vi "Log Result.vi"(8 "error in (no error)":errorcluster, 10 "Result":refnum<class "Acquired Result.lvclass">, 11 "Process Controller in":refnum<class "Process Controller.lvclass">) -> (0 "error out":errorcluster, 2 "Result out":refnum<class "Acquired Result.lvclass">, 3 "Process Controller out":refnum<class "Process Controller.lvclass">)   [LabVIEW 2016, in "Process Controller.lvclass"]
uses:
  Process Controller.lvclass
  C:/github/LabActor/Template Module/Template Module.lvclass
  C:/github/LabActor/Worker/Worker.lvclass
  NHMFL_Core/Libraries/Instruments/Results/Acquired Result/Acquired Result.lvclass
  Template Module/Template Module.lvclass/Template Module.ctl
  Process Controller.lvclass/Process Controller.ctl
  Worker/Worker.lvclass/Worker.ctl
  Loggers/Logger Messages/Log Result Msg/Log Result Msg.lvclass/Log Result Msg.ctl
  <vilib>/ActorFramework/Message Enqueuer/Message Enqueuer.lvclass/Message Enqueuer.ctl
  Template Module/Write Logger.vi
  Template Module/Read Logger.vi
  Read Timestamp data points.vi
  Worker/Read Use buffered logger.vi
  Worker/Read Remote logger launched.vi
  Worker/Read Logger Enqueuer.vi
  <vilib>/ActorFramework/Message Enqueuer/Enqueue.vi
  Loggers/Logger Messages/Log Result Msg/Log Result Msg.lvclass
  C:/Program Files/National Instruments/LabVIEW 2016/vi.lib/ActorFramework/Message/Message.lvclass
  <vilib>/ActorFramework/Message Priority Queue/Priority Enqueue.vi
  Loggers/Logger/Logger.lvclass
  <vilib>/ActorFramework/Message Enqueuer/Message Enqueuer.lvclass
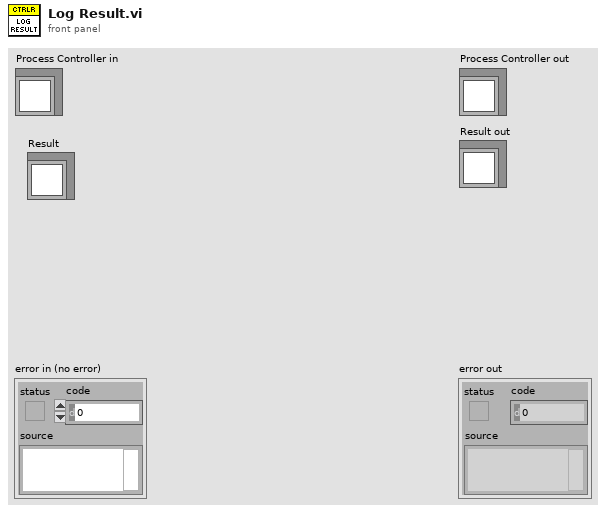
[diagram p1: front panel]
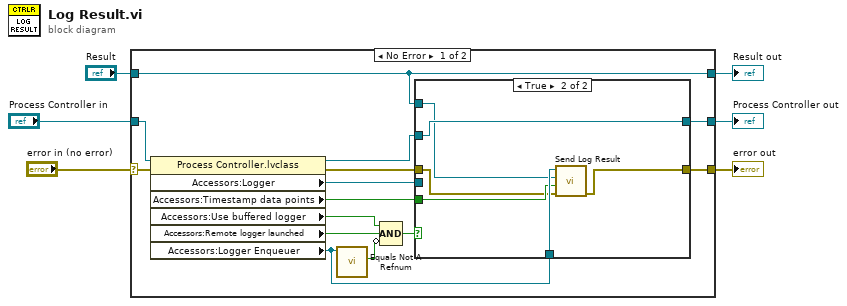
[diagram p0: block diagram]
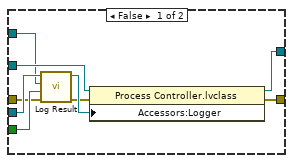
[diagram p2: hidden frame]
diagram:
  n1 = case shown="No Error" "error in (no error)" {
    selector: "error in (no error)" -> [w20 w38]
    tunnel: [w19 w38] -> w5
    tunnel: [w16 w37] -> w3
    tunnel: "Process Controller in" -> [w17 w37]
    tunnel: "Result" -> [w14 w36]
    tunnel: [w14 w36] -> w1
    frame No Error {
      n2 = property class="Process Controller.lvclass"(reference=w17, error in=w20) -> (reference out=w18:refnum<class "Process Controller.lvclass">, error out=w12:errorcluster, "Accessors:Logger"=w15:refnum<class "Logger.lvclass">, "Accessors:Timestamp data points"=w13:bool, "Accessors:Use buffered logger"=w10:bool, "Accessors:Remote logger launched"=w9:bool, "Accessors:Logger Enqueuer"=w7:refnum<class "Message Enqueuer.lvclass">)
      n3 = call <vilib>:"Equals Not A Refnum.vi"("Message Enqueuer"=w7) -> ("Not a refnum?"=w11:bool)  [unwired: 10 in]
      n4 = Compound Arithmetic op=AND(w10, w9, invert w11) -> (w8:bool)
      n5 = case shown="True" w8 {
        tunnel: [w29 w30] -> w19
        tunnel: w18 -> [w28 w35]
        tunnel: [w27 w35] -> w16
        tunnel: w15 -> [w26 _]
        tunnel: w14 -> [w24 w33]
        tunnel: w13 -> [w23 w32]
        tunnel: w12 -> [w22 w31]
        tunnel: w7 -> [_ w34]
        frame False {
          n6 = call-dynamic "Log Result.vi"("error in (no error)"=w22, "Timestamp data points"=w23, "Result"=w24, "Logger in"=w26) -> ("error out"=w21:errorcluster, "Logger out"=w25:refnum<class "Logger.lvclass">)  [unwired: 6 in]
          n7 = property class="Process Controller.lvclass"(reference=w28, error in=w21, "Accessors:Logger"=w25) -> (reference out=w27:refnum<class "Process Controller.lvclass">, error out=w29:errorcluster)
        }
        frame True {
          n8 = call "Send Log Result.vi"("error in (no error)"=w31, "Timestamp data points"=w32, "Result"=w33, "Message Enqueuer"=w34) -> ("error out"=w30:errorcluster)  [unwired: 6 in, 1 out]
        }
      }
    }
    frame Error {
    }
  }
  "error out" <- w5
  "Process Controller out" <- w3
  "Result out" <- w1
